vi "test_read-nmea-data2.vi"() -> ()   [LabVIEW 2019] (continued)
205,26,72,03,209,,1*76\n\t\n15:11:25.53\tF9P\t$GLGSV,2,2,08,77,01,326,,84,20,122,08,85,70,065,25,86,36,330,,1*74\n\t\n15:11:25.55\tF9P\t$GLGSV,2,1,08,69,12,031,,70,72,041,,71,51,205,24,72,03,209,,3*76\n\t\n15:11:25.57\tF9P\t$GLGSV,2,2,08,77,01,326,,84,20,122,18,85,70,065,21,86,36,330,,3*73\n\t\n15:11:25.59\tF9P\t$GAGSV,2,1,08,02,08,297,09,04,66,118,29,09,32,193,26,11,71,358,24,7*79\n\t\n15:11:25.61\tF9P\t$GAGSV,2,2,08,12,40,102,26,19,26,045,17,25,09,249,,36,26,308,35,7*7D\n\t\n15:11:25.63\tF9P\t$GAGSV,2,1,08,02,08,297,,04,66,118,27,09,32,193,,11,71,358,,2*79\n\t\n15:11:25.65\tF9P\t$GAGSV,2,2,08,12,40,102,,19,26,045,,25,09,249,,36,26,308,,2*7C\n\t\n15:11:25.67\tF9P\t$GBGSV,1,1,03,11,50,132,26,14,87,127,23,33,60,219,24,1*41\n\t\n15:11:25.69\tF9P\t$GBGSV,1,1,03,11,50,132,30,14,87,127,,33,60,219,,3*43\n\t\n15:11:25.71\tF9P\t$GNGLL,3723.53368,N,12656.90596,E,061127.00,A,A*7F\n\t\n15:11:25.73\tF9P\t\t\n15:11:25.75\tF9P\t\t\n15:11:25.77\tF9P\t\t\n15:11:25.79\tF9P\t\t\n15:11:25.81\tF9P\t\t\n15:11:25.83\tF9P\t\t\n15:11:25.85\tF9P\t\t\n15:11:25.87\tF9P\t\t\n15:11:25.89\tF9P\t\t\n15:11:25.91\tF9P\t\t\n15:11:25.93\tF9P\t\t\n15:11:25.95\tF9P\t\t\n15:11:25.97\tF9P\t\t\n15:11:25.99\tF9P\t\t\n15:11:26.01\tF9P\t\t\n15:11:26.03\tF9P\t\t\n15:11:26.05\tF9P\t\t\n15:11:26.07\tF9P\t\t\n15:11:26.09\tF9P\t\t\n15:11:26.11\tF9P\t\t\n15:11:26.13\tF9P\t\t\n15:11:26.15\tF9P\t\t\n15:11:26.17\tF9P\t\t\n15:11:26.19\tF9P\t\t\n15:11:26.21\tF9P\t\t\n15:11:26.23\tF9P\t\t\n15:11:26.25\tF9P\t$GNRMC,061128.00,A,3723.53331,N,12656.90644,E,1.898,132.24,250720,,,A,V*01\n\t\n15:11:26.27\tF9P\t$GNVTG,132.24,T,,M,1.898,N,3.516,K,A*2C\n\t\n15:11:26.29\tF9P\t$GNGGA,061128.00,3723.53331,N,12656.90644,E,1,12,0.72,35.9,M,18.5,M,,*70\n\t\n15:11:26.32\tF9P\t$GNGSA,A,3,12,06,19,05,17,09,04,02,,,,,1.36,0.72,1.15,1*04\n\t\n15:11:26.34\tF9P\t$GNGSA,A,3,85,71,84,,,,,,,,,,1.36,0.72,1.15,2*01\n\t\n15:11:26.36\tF9P\t$GNGSA,A,3,36,19,11,04,09,12,,,,,,,1.36,0.72,1.15,3*04\n\t\n15:11:26.38\tF9P\t$GNGSA,A,3,14,11,33,,,,,,,,,,1.36,0.72,1.15,4*05\n\t\n15:11:26.40\tF9P\t$GPGSV,3,1,09,02,54,318,30,04,18,044,18,05,37,247,19,06,64,047,30,1*6D\n\t\n15:11:26.42\tF9P\t$GPGSV,3,2,09,09,45,074,31,12,24,277,22,17,33,153,28,19,53,157,31,1*66\n\t\n15:11:26.44\tF9P\t$GPGSV,3,3,09,25,12,307,16,1*5A\n\t\n15:11:26.46\tF9P\t$GPGSV,3,1,09,02,54,318,,04,18,044,,05,37,247,19,06,64,047,29,6*68\n\t\n15:11:26.48\tF9P\t$GPGSV,3,2,09,09,45,074,31,12,24,277,,17,33,153,23,19,53,157,,6*68\n\t\n15:11:26.50\tF9P\t$GPGSV,3,3,09,25,12,307,,6*5A\n\t\n15:11:26.52\tF9P\t$GLGSV,2,1,08,69,12,031,,70,72,041,,71,51,205,26,72,03,209,,1*76\n\t\n15:11:26.54\tF9P\t$GLGSV,2,2,08,77,01,326,,84,20,122,10,85,70,065,37,86,36,330,,1*7E\n\t\n15:11:26.56\tF9P\t$GLGSV,2,1,08,69,12,031,,70,72,041,,71,51,205,24,72,03,209,,3*76\n\t\n15:11:26.58\tF9P\t$GLGSV,2,2,08,77,01,326,,84,20,122,20,85,70,065,22,86,36,330,,3*7B\n\t\n15:11:26.60\tF9P\t$GAGSV,2,1,08,02,08,297,09,04,66,118,28,09,32,193,26,11,71,358,24,7*78\n\t\n15:11:26.62\tF9P\t$GAGSV,2,2,08,12,40,102,24,19,26,045,14,25,09,249,,36,26,308,30,7*79\n\t\n15:11:26.64\tF9P\t$GAGSV,2,1,08,02,08,297,,04,66,118,27,09,32,193,,11,71,358,,2*79\n\t\n15:11:26.66\tF9P\t$GAGSV,2,2,08,12,40,102,,19,26,045,,25,09,249,,36,26,308,,2*7C\n\t\n15:11:26.68\tF9P\t$GBGSV,1,1,03,11,50,132,28,14,87,127,23,33,60,219,26,1*4D\n\t\n15:11:26.70\tF9P\t$GBGSV,1,1,03,11,50,132,,14,87,127,,33,60,219,,3*40\n\t\n15:11:26.72\tF9P\t$GNGLL,3723.53331,N,12656.90644,E,061128.00,A,A*70\n\t\n15:11:26.74\tF9P\t\t\n15:11:26.76\tF9P\t\t\n15:11:26.78\tF9P\t\t\n15:11:26.80\tF9P\t\t\n15:11:26.82\tF9P\t\t\n15:11:26.84\tF9P\t\t\n15:11:26.86\tF9P\t\t\n15:11:26.88\tF9P\t\t\n15:11:26.90\tF9P\t\t\n15:11:26.92\tF9P\t\t\n15:11:26.94\tF9P\t\t\n15:11:26.96\tF9P\t\t\n15:11:26.98\tF9P\t\t\n15:11:27.00\tF9P\t\t\n15:11:27.02\tF9P\t\t\n15:11:27.04\tF9P\t\t\n15:11:27.06\tF9P\t\t\n15:11:27.08\tF9P\t\t\n15:11:27.10\tF9P\t\t\n15:11:27.12\tF9P\t\t\n15:11:27.14\tF9P\t\t\n15:11:27.16\tF9P\t\t\n15:11:27.18\tF9P\t\t\n15:11:27.20\tF9P\t\t\n15:11:27.22\tF9P\t\t\n15:11:27.24\tF9P\t\t\n15:11:27.26\tF9P\t$GNRMC,061129.00,A,3723.53261,N,12656.90690,E,1.894,136.64,250720,,,A,V*01\n\t\n15:11:27.28\tF9P\t$GNVTG,136.64,T,,M,1.894,N,3.507,K,A*20\n\t\n15:11:27.30\tF9P\t$GNGGA,061129.00,3723.53261,N,12656.90690,E,1,12,0.72,36.2,M,18.5,M,,*74\n\t\n15:11:27.32\tF9P\t$GNGSA,A,3,12,06,19,05,17,09,02,,,,,,1.36,0.72,1.15,1*00\n\t\n15:11:27.34\tF9P\t$GNGSA,A,3,85,71,84,,,,,,,,,,1.36,0.72,1.15,2*01\n\t\n15:11:27.36\tF9P\t$GNGSA,A,3,36,19,11,04,09,12,,,,,,,1.36,0.72,1.15,3*04\n\t\n15:11:27.38\tF9P\t$GNGSA,A,3,14,11,33,,,,,,,,,,1.36,0.72,1.15,4*05\n\t\n15:11:27.40\tF9P\t$GPGSV,3,1,09,02,54,318,25,04,18,044,,05,37,247,22,06,64,047,29,1*60\n\t\n15:11:27.42\tF9P\t$GPGSV,3,2,09,09,45,074,32,12,24,277,22,17,33,153,32,19,53,157,39,1*66\n\t\n15:11:27.44\tF9P\t$GPGSV,3,3,09,25,12,307,17,1*5B\n\t\n15:11:27.46\tF9P\t$GPGSV,3,1,09,02,54,318,,04,18,044,,05,37,247,19,06,64,047,32,6*62\n\t\n15:11:27.48\tF9P\t$GPGSV,3,2,09,09,45,074,28,12,24,277,,17,33,153,24,19,53,157,,6*67\n\t\n15:11:27.50\tF9P\t$GPGSV,3,3,09,25,12,307,,6*5A\n\t\n15:11:27.52\tF9P\t$GLGSV,2,1,08,69,12,031,,70,72,041,,71,51,205,37,72,03,209,,1*76\n\t\n15:11:27.54\tF9P\t$GLGSV,2,2,08,77,01,326,,84,20,122,10,85,70,065,30,86,36,330,,1*79\n\t\n15:11:27.56\tF9P\t$GLGSV,2,1,08,69,12,031,,70,72,041,,71,51,205,31,72,03,209,,3*72\n\t\n15:11:27.58\tF9P\t$GLGSV,2,2,08,77,01,326,,84,20,122,19,85,70,065,30,86,36,330,,3*72\n\t\n15:11:27.60\tF9P\t$GAGSV,2,1,08,02,08,297,09,04,66,118,26,09,32,193,31,11,71,358,24,7*70\n\t\n15:11:27.62\tF9P\t$GAGSV,2,2,08,12,40,102,24,19,26,045,12,25,09,249,,36,26,308,28,7*76\n\t\n15:11:27.64\tF9P\t$GAGSV,2,1,08,02,08,297,,04,66,118,27,09,32,193,,11,71,358,,2*79\n\t\n15:11:27.66\tF9P\t$GAGSV,2,2,08,12,40,102,,19,26,045,,25,09,249,,36,26,308,,2*7C\n\t\n15:11:27.68\tF9P\t$GBGSV,1,1,03,11,50,132,27,14,87,127,31,33,60,219,31,1*47\n\t\n15:11:27.70\tF9P\t$GBGSV,1,1,03,11,50,132,27,14,87,127,,33,60,219,,3*45\n\t\n15:11:27.72\tF9P\t$GNGLL,3723.53261,N,12656.90690,E,061129.00,A,A*7C\n\t\n15:11:27.74\tF9P\t\t\n15:11:27.76\tF9P\t\t\n15:11:27.78\tF9P\t\t\n15:11:27.80\tF9P\t\t\n15:11:27.82\tF9P\t\t\n15:11:27.84\tF9P\t\t\n15:11:27.86\tF9P\t\t\n15:11:27.88\tF9P\t\t\n15:11:27.90\tF9P\t\t\n15:11:27.92\tF9P\t\t\n15:11:27.94\tF9P\t\t\n15:11:27.96\tF9P\t\t\n15:11:27.98\tF9P\t\t\n15:11:28.00\tF9P\t\t\n15:11:28.02\tF9P\t\t\n15:11:28.04\tF9P\t\t\n15:11:28.06\tF9P\t\t\n15:11:28.08\tF9P\t\t\n15:11:28.10\tF9P\t\t\n15:11:28.12\tF9P\t\t\n15:11:28.14\tF9P\t\t\n15:11:28.16\tF9P\t\t\n15:11:28.18\tF9P\t\t\n15:11:28.20\tF9P\t\t\n15:11:28.22\tF9P\t\t\n15:11:28.24\tF9P\t\t\n15:11:28.26\tF9P\t$GNRMC,061130.00,A,3723.53163,N,12656.90719,E,2.333,141.66,250720,,,A,V*0F\n\t\n15:11:28.28\tF9P\t$GNVTG,141.66,T,,M,2.333,N,4.322,K,A*21\n\t\n15:11:28.30\tF9P\t$GNGGA,061130.00,3723.53163,N,12656.90719,E,1,12,0.72,35.9,M,18.5,M,,*75\n\t\n15:11:28.32\tF9P\t$GNGSA,A,3,12,06,19,05,17,09,02,,,,,,1.36,0.72,1.15,1*00\n\t\n15:11:28.34\tF9P\t$GNGSA,A,3,85,71,84,,,,,,,,,,1.36,0.72,1.15,2*01\n\t\n15:11:28.36\tF9P\t$GNGSA,A,3,36,19,11,04,09,12,,,,,,,1.36,0.72,1.15,3*04\n\t\n15:11:28.38\tF9P\t$GNGSA,A,3,14,11,33,,,,,,,,,,1.36,0.72,1.15,4*05\n\t\n15:11:28.40\tF9P\t$GPGSV,3,1,09,02,54,318,32,04,18,044,,05,37,247,25,06,64,047,30,1*69\n\t\n15:11:28.42\tF9P\t$GPGSV,3,2,09,09,45,074,27,12,24,277,23,17,33,153,39,19,53,157,29,1*69\n\t\n15:11:28.44\tF9P\t$GPGSV,3,3,09,25,12,307,16,1*5A\n\t\n15:11:28.46\tF9P\t$GPGSV,3,1,09,02,54,318,,04,18,044,,05,37,247,17,06,64,047,27,6*68\n\t\n15:11:28.48\tF9P\t$GPGSV,3,2,09,09,45,074,26,12,24,277,,17,33,153,24,19,53,157,,6*69\n\t\n15:11:28.50\tF9P\t$GPGSV,3,3,09,25,12,307,,6*5A\n\t\n15:11:28.52\tF9P\t$GLGSV,2,1,08,69,12,031,,70,72,041,,71,51,205,32,72,03,209,,1*73\n\t\n15:11:28.54\tF9P\t$GLGSV,2,2,08,77,01,326,,84,20,122,16,85,70,065,24,86,36,330,,1*7A\n\t\n15:11:28.56\tF9P\t$GLGSV,2,1,08,69,12,031,,70,72,041,,71,51,205,24,72,03,209,,3*76\n\t\n15:11:28.58\tF9P\t$GLGSV,2,2,08,77,01,326,,84,20,122,17,85,70,065,23,86,36,330,,3*7E\n\t\n15:11:28.60\tF9P\t$GAGSV,2,1,08,02,08,297,11,04,66,118,30,09,32,193,26,11,71,358,23,7*7F\n\t\n15:11:28.62\tF9P\t$GAGSV,2,2,08,12,40,102,24,19,26,045,10,25,09,249,,36,26,308,29,7*75\n\t\n15:11:28.64\tF9P\t$GAGSV,2,1,08,02,08,297,,04,66,118,30,09,32,193,32,11,71,358,,2*7E\n\t\n15:11:28.66\tF9P\t$GAGSV,2,2,08,12,40,102,26,19,26,045,,25,09,249,,36,26,308,,2*78\n\t\n15:11:28.68\tF9P\t$GBGSV,1,1,03,11,50,132,27,14,87,127,26,33,60,219,36,1*46\n\t\n15:11:28.70\tF9P\t$GBGSV,1,1,03,11,50,132,27,14,87,127,,33,60,219,,3*45\n\t\n15:11:28.72\tF9P\t$GNGLL,3723.53163,N,12656.90719,E,061130.00,A,A*75\n\t\n15:11:28.74\tF9P\t\t\n15:11:28.76\tF9P\t\t\n15:11:28.78\tF9P\t\t\n15:11:28.80\tF9P\t\t\n15:11:28.82\tF9P\t\t\n15:11:28.84\tF9P\t\t\n15:11:28.86\tF9P\t\t\n15:11:28.88\tF9P\t\t\n15:11:28.90\tF9P\t\t\n15:11:28.92\tF9P\t\t\n15:11:28.94\tF9P\t\t\n15:11:28.96\tF9P\t\t\n15:11:28.98\tF9P\t\t\n15:11:29.00\tF9P\t\t\n15:11:29.02\tF9P\t\t\n15:11:29.04\tF9P\t\t\n15:11:29.06\tF9P\t\t\n15:11:29.08\tF9P\t\t\n15:11:29.10\tF9P\t\t\n15:11:29.12\tF9P\t\t\n15:11:29.14\tF9P\t\t\n15:11:29.16\tF9P\t\t\n15:11:29.18\tF9P\t\t\n15:11:29.20\tF9P\t\t\n15:11:29.22\tF9P\t\t\n15:11:29.24\tF9P\t$GNRMC,061131.00,A,3723.53091,N,12656.90746,E,2.306,147.77,250720,,,A,V*08\n\t\n15:11:29.26\tF9P\t$GNVTG,147.77,T,,M,2.306,N,4.271,K,A*26\n\t\n15:11:29.28\tF9P\t$GNGGA,061131.00,3723.53091,N,12656.90746,E,1,12,0.79,35.8,M,18.5,M,,*78\n\t\n15:11:29.30\tF9P\t$GNGSA,A,3,12,06,19,05,17,09,02,,,,,,1.50,0.79,1.27,1*0A\n\t\n15:11:29.32\tF9P\t$GNGSA,A,3,85,71,84,,,,,,,,,,1.50,0.79,1.27,2*0B\n\t\n15:11:29.34\tF9P\t$GNGSA,A,3,36,19,11,04,09,12,,,,,,,1.50,0.79,1.27,3*0E\n\t\n15:11:29.36\tF9P\t$GNGSA,A,3,14,11,33,,,,,,,,,,1.50,0.79,1.27,4*0F\n\t\n15:11:29.38\tF9P\t$GPGSV,3,1,09,02,54,318,31,04,18,044,18,05,37,247,31,06,64,047,34,1*62\n\t\n15:11:29.40\tF9P\t$GPGSV,3,2,09,09,45,074,31,12,24,277,23,17,33,153,34,19,53,157,32,1*69\n\t\n15:11:29.42\tF9P\t$GPGSV,3,3,09,25,12,307,15,1*59\n\t\n15:11:29.44\tF9P\t$GPGSV,3,1,09,02,54,318,,04,18,044,,05,37,247,15,06,64,047,25,6*68\n\t\n15:11:29.46\tF9P\t$GPGSV,3,2,09,09,45,074,27,12,24,277,,17,33,153,34,19,53,157,,6*69\n\t\n15:11:29.48\tF9P\t$GPGSV,3,3,09,25,12,307,,6*5A\n\t\n15:11:29.50\tF9P\t$GLGSV,2,1,08,69,12,031,,70,72,041,,71,51,205,32,72,03,209,,1*73\n\t\n15:11:29.52\tF9P\t$GLGSV,2,2,08,77,01,326,,84,20,122,10,85,70,065,30,86,36,330,,1*79\n\t\n15:11:29.54\tF9P\t$GLGSV,2,1,08,69,12,031,,70,72,041,,71,51,205,24,72,03,209,,3*76\n\t\n15:11:29.56\tF9P\t$GLGSV,2,2,08,77,01,326,,84,20,122,13,85,70,065,22,86,36,330,,3*7B\n\t\n15:11:29.58\tF9P\t$GAGSV,2,1,08,02,08,297,09,04,66,118,30,09,32,193,35,11,71,358,25,7*72\n\t\n15:11:29.60\tF9P\t$GAGSV,2,2,08,12,40,102,24,19,26,045,15,25,09,249,,36,26,308,31,7*79\n\t\n15:11:29.62\tF9P\t$GAGSV,2,1,08,02,08,297,,04,66,118,30,09,32,193,26,11,71,358,,2*7B\n\t\n15:11:29.64\tF9P\t$GAGSV,2,2,08,12,40,102,25,19,26,045,,25,09,249,,36,26,308,,2*7B\n\t\n15:11:29.66\tF9P\t$GBGSV,1,1,03,11,50,132,26,14,87,127,26,33,60,219,33,1*42\n\t\n15:11:29.68\tF9P\t$GBGSV,1,1,03,11,50,132,,14,87,127,,33,60,219,,3*40\n\t\n15:11:29.70\tF9P\t$GNGLL,3723.53091,N,12656.90746,E,061131.00,A,A*72\n\t\n15:11:29.72\tF9P\t\t\n15:11:29.74\tF9P\t\t\n15:11:29.76\tF9P\t\t\n15:11:29.78\tF9P\t\t\n15:11:29.80\tF9P\t\t\n15:11:29.82\tF9P\t\t\n15:11:29.84\tF9P\t\t\n15:11:29.86\tF9P\t\t\n15:11:29.88\tF9P\t\t\n15:11:29.90\tF9P\t\t\n15:11:29.92\tF9P\t\t\n15:11:29.94\tF9P\t\t\n15:11:29.96\tF9P\t\t\n15:11:29.98\tF9P\t\t\n15:11:30.00\tF9P\t\t\n15:11:30.02\tF9P\t\t\n15:11:30.04\tF9P\t\t\n15:11:30.06\tF9P\t\t\n15:11:30.08\tF9P\t\t\n15:11:30.10\tF9P\t\t\n15:11:30.12\tF9P\t\t\n15:11:30.14\tF9P\t\t\n15:11:30.16\tF9P\t\t\n15:11:30.18\tF9P\t\t\n15:11:30.20\tF9P\t\t\n15:11:30.22\tF9P\t\t\n15:11:30.24\tF9P\t\t\n15:11:30.26\tF9P\t$GNRMC,061132.00,A,3723.53020,N,12656.90826,E,2.392,137.11,250720,,,A,V*02\n\t\n15:11:30.28\tF9P\t$GNVTG,137.11,T,,M,2.392,N,4.430,K,A*2F\n\t\n15:11:30.30\tF9P\t$GNGGA,061132.00,3723.53020,N,12656.90826,E,1,12,0.68,35.3,M,18.5,M,,*73\n\t\n15:11:30.32\tF9P\t$GNGSA,A,3,12,06,19,05,17,09,02,,,,,,1.27,0.68,1.08,1*07\n\t\n15:11:30.34\tF9P\t$GNGSA,A,3,85,71,84,,,,,,,,,,1.27,0.68,1.08,2*06\n\t\n15:11:30.36\tF9P\t$GNGSA,A,3,36,19,11,04,09,12,,,,,,,1.27,0.68,1.08,3*03\n\t\n15:11:30.38\tF9P\t$GNGSA,A,3,14,11,33,,,,,,,,,,1.27,0.68,1.08,4*02\n\t\n15:11:30.40\tF9P\t$GPGSV,3,1,09,02,54,318,35,04,18,044,19,05,37,247,24,06,64,047,39,1*6E\n\t\n15:11:30.42\tF9P\t$GPGSV,3,2,09,09,45,074,33,12,24,277,29,17,33,153,38,19,53,157,36,1*69\n\t\n15:11:30.44\tF9P\t$GPGSV,3,3,09,25,12,307,16,1*5A\n\t\n15:11:30.46\tF9P\t$GPGSV,3,1,09,02,54,318,,04,18,044,,05,37,247,,06,64,047,23,6*6A\n\t\n15:11:30.48\tF9P\t$GPGSV,3,2,09,09,45,074,27,12,24,277,,17,33,153,22,19,53,157,,6*6E\n\t\n15:11:30.50\tF9P\t$GPGSV,3,3,09,25,12,307,,6*5A\n\t\n15:11:30.52\tF9P\t$GLGSV,2,1,08,69,12,031,,70,72,041,,71,51,205,39,72,03,209,,1*78\n\t\n15:11:30.54\tF9P\t$GLGSV,2,2,08,77,01,326,,84,20,122,11,85,70,065,30,86,36,330,,1*78\n\t\n15:11:30.56\tF9P\t$GLGSV,2,1,08,69,12,031,,70,72,041,,71,51,205,31,72,03,209,,3*72\n\t\n15:11:30.58\tF9P\t$GLGSV,2,2,08,77,01,326,,84,20,122,16,85,70,065,21,86,36,330,,3*7D\n\t\n15:11:30.60\tF9P\t$GAGSV,2,1,08,02,08,297,11,04,66,118,30,09,32,193,28,11,71,358,21,7*73\n\t\n15:11:30.62\tF9P\t$GAGSV,2,2,08,12,40,102,23,19,26,045,10,25,09,249,,36,26,308,32,7*78\n\t\n15:11:30.64\tF9P\t$GAGSV,2,1,08,02,08,297,,04,66,118,25,09,32,193,25,11,71,358,,2*7C\n\t\n15:11:30.66\tF9P\t$GAGSV,2,2,08,12,40,102,25,19,26,045,,25,09,249,,36,26,308,,2*7B\n\t\n15:11:30.68\tF9P\t$GBGSV,1,1,03,11,50,132,26,14,87,127,30,33,60,219,35,1*43\n\t\n15:11:30.70\tF9P\t$GBGSV,1,1,03,11,50,132,27,14,87,127,,33,60,219,,3*45\n\t\n15:11:30.72\tF9P\t$GNGLL,3723.53020,N,12656.90826,E,061132.00,A,A*72\n\t\n15:11:30.74\tF9P\t\t\n15:11:30.76\tF9P\t\t\n15:11:30.78\tF9P\t\t\n15:11:30.80\tF9P\t\t\n15:11:30.82\tF9P\t\t\n15:11:30.84\tF9P\t\t\n15:11:30.86\tF9P\t\t\n15:11:30.88\tF9P\t\t\n15:11:30.90\tF9P\t\t\n15:11:30.92\tF9P\t\t\n15:11:30.94\tF9P\t\t\n15:11:30.96\tF9P\t\t\n15:11:30.98\tF9P\t\t\n15:11:31.00\tF9P\t\t\n15:11:31.02\tF9P\t\t\n15:11:31.04\tF9P\t\t\n15:11:31.06\tF9P\t\t\n15:11:31.08\tF9P\t\t\n15:11:31.10\tF9P\t\t\n15:11:31.12\tF9P\t\t\n15:11:31.14\tF9P\t\t\n15:11:31.16\tF9P\t\t\n15:11:31.18\tF9P\t\t\n15:11:31.20\tF9P\t\t\n15:11:31.22\tF9P\t\t\n15:11:31.24\tF9P\t$GNRMC,061133.00,A,3723.52963,N,12656.90859,E,2.005,138.73,250720,,,A,V*02\n\t\n15:11:31.26\tF9P\t$GNVTG,138.73,T,,M,2.005,N,3.714,K,A*2B\n\t\n15:11:31.28\tF9P\t$GNGGA,061133.00,3723.52963,N,12656.90859,E,1,12,0.72,35.3,M,18.5,M,,*7E\n\t\n15:11:31.30\tF9P\t$GNGSA,A,3,12,06,19,05,17,09,02,,,,,,1.36,0.72,1.15,1*00\n\t\n15:11:31.32\tF9P\t$GNGSA,A,3,85,71,84,,,,,,,,,,1.36,0.72,1.15,2*01\n\t\n15:11:31.34\tF9P\t$GNGSA,A,3,36,19,11,04,09,12,,,,,,,1.36,0.72,1.15,3*04\n\t\n15:11:31.36\tF9P\t$GNGSA,A,3,14,11,33,,,,,,,,,,1.36,0.72,1.15,4*05\n\t\n15:11:31.38\tF9P\t$GPGSV,3,1,09,02,54,318,35,04,18,044,18,05,37,247,24,06,64,047,38,1*6E\n\t\n15:11:31.40\tF9P\t$GPGSV,3,2,09,09,45,074,32,12,24,277,27,17,33,153,35,19,53,157,33,1*6E\n\t\n15:11:31.42\tF9P\t$GPGSV,3,3,09,25,12,307,17,1*5B\n\t\n15:11:31.44\tF9P\t$GPGSV,3,1,09,02,54,318,,04,18,044,,05,37,247,,06,64,047,21,6*68\n\t\n15:11:31.46\tF9P\t$GPGSV,3,2,09,09,45,074,27,12,24,277,,17,33,153,22,19,53,157,,6*6E\n\t\n15:11:31.48\tF9P\t$GPGSV,3,3,09,25,12,307,,6*5A\n\t\n15:11:31.50\tF9P\t$GLGSV,2,1,08,69,12,031,,70,71,039,,71,51,205,32,72,03,209,,1*7F\n\t\n15:11:31.52\tF9P\t$GLGSV,2,2,08,77,01,326,,84,20,122,17,85,70,065,30,86,36,330,,1*7E\n\t\n15:11:31.54\tF9P\t$GLGSV,2,1,08,69,12,031,,70,71,039,,71,51,205,27,72,03,209,,3*79\n\t\n15:11:31.56\tF9P\t$GLGSV,2,2,08,77,01,326,,84,20,122,15,85,70,065,22,86,36,330,,3*7D\n\t\n15:11:31.58\tF9P\t$GAGSV,2,1,08,02,08,297,10,04,66,118,29,09,32,193,31,11,71,358,29,7*7A\n\t\n15:11:31.60\tF9P\t$GAGSV,2,2,08,12,40,102,23,19,26,045,10,25,09,249,,36,26,308,37,7*7D\n\t\n15:11:31.62\tF9P\t$GAGSV,2,1,08,02,08,297,,04,66,118,24,09,32,193,25,11,71,358,,2*7D\n\t\n15:11:31.64\tF9P\t$GAGSV,2,2,08,12,40,102,26,19,26,045,,25,09,249,,36,26,308,,2*78\n\t\n15:11:31.66\tF9P\t$GBGSV,1,1,03,11,50,132,31,14,87,127,25,33,60,219,31,1*45\n\t\n15:11:31.68\tF9P\t$GBGSV,1,1,03,11,50,132,26,14,87,127,,33,60,219,,3*44\n\t\n15:11:31.70\tF9P\t$GNGLL,3723.52963,N,12656.90859,E,061133.00,A,A*74\n\t\n15:11:31.72\tF9P\t\t\n15:11:31.74\tF9P\t\t\n15:11:31.76\tF9P\t\t\n15:11:31.78\tF9P\t\t\n15:11:31.80\tF9P\t\t\n15:11:31.82\tF9P\t\t\n15:11:31.84\tF9P\t\t\n15:11:31.86\tF9P\t\t\n15:11:31.88\tF9P\t\t\n15:11:31.90\tF9P\t\t\n15:11:31.92\tF9P\t\t\n15:11:31.94\tF9P\t\t\n15:11:31.96\tF9P\t\t\n15:11:31.98\tF9P\t\t\n15:11:32.00\tF9P\t\t\n15:11:32.02\tF9P\t\t\n15:11:32.04\tF9P\t\t\n15:11:32.06\tF9P\t\t\n15:11:32.08\tF9P\t\t\n15:11:32.10\tF9P\t\t\n15:11:32.12\tF9P\t\t\n15:11:32.14\tF9P\t\t\n15:11:32.16\tF9P\t\t\n15:11:32.18\tF9P\t\t\n15:11:32.20\tF9P\t\t\n15:11:32.22\tF9P\t\t\n15:11:32.24\tF9P\t\t\n15:11:32.26\tF9P\t$GNRMC,061134.00,A,3723.52948,N,12656.90973,E,2.314,119.55,250720,,,A,V*01\n\t\n15:11:32.28\tF9P\t$GNVTG,119.55,T,,M,2.314,N,4.285,K,A*25\n\t\n15:11:32.30\tF9P\t$GNGGA,061134.00,3723.52948,N,12656.90973,E,1,12,0.72,34.5,M,18.5,M,,*7E\n\t\n15:11:32.32\tF9P\t$GNGSA,A,3,12,06,19,05,17,09,02,,,,,,1.36,0.72,1.15,1*00\n\t\n15:11:32.34\tF9P\t$GNGSA,A,3,85,71,84,,,,,,,,,,1.36,0.72,1.15,2*01\n\t\n15:11:32.36\tF9P\t$GNGSA,A,3,36,19,11,04,09,12,,,,,,,1.36,0.72,1.15,3*04\n\t\n15:11:32.38\tF9P\t$GNGSA,A,3,14,11,33,,,,,,,,,,1.36,0.72,1.15,4*05\n\t\n15:11:32.40\tF9P\t$GPGSV,3,1,09,02,54,318,39,04,18,044,27,05,37,247,25,06,64,047,47,1*67\n\t\n15:11:32.42\tF9P\t$GPGSV,3,2,09,09,45,074,43,12,24,277,28,17,33,153,36,19,53,157,35,1*62\n\t\n15:11:32.44\tF9P\t$GPGSV,3,3,09,25,12,307,18,1*54\n\t\n15:11:32.46\tF9P\t$GPGSV,3,1,09,02,54,318,,04,18,044,,05,37,247,,06,64,047,20,6*69\n\t\n15:11:32.48\tF9P\t$GPGSV,3,2,09,09,45,074,25,12,24,277,,17,33,153,23,19,53,157,,6*6D\n\t\n15:11:32.50\tF9P\t$GPGSV,3,3,09,25,12,307,,6*5A\n\t\n15:11:32.52\tF9P\t$GLGSV,2,1,08,69,12,031,,70,71,039,,71,52,205,34,72,03,209,,1*7A\n\t\n15:11:32.54\tF9P\t$GLGSV,2,2,08,77,01,326,,84,20,122,15,85,70,065,37,86,36,330,,1*7B\n\t\n15:11:32.56\tF9P\t$GLGSV,2,1,08,69,12,031,,70,71,039,,71,52,205,25,72,03,209,,3*78\n\t\n15:11:32.58\tF9P\t$GLGSV,2,2,08,77,01,326,,84,20,122,15,85,70,065,23,86,36,330,,3*7C\n\t\n15:11:32.60\tF9P\t$GAGSV,2,1,08,02,08,297,07,04,66,118,32,09,32,193,27,11,71,358,34,7*7D\n\t\n15:11:32.62\tF9P\t$GAGSV,2,2,08,12,40,102,30,19,26,045,12,25,09,249,,36,26,308,30,7*7A\n\t\n15:11:32.64\tF9P\t$GAGSV,2,1,08,02,08,297,,04,66,118,,09,32,193,23,11,71,358,,2*7D\n\t\n15:11:32.66\tF9P\t$GAGSV,2,2,08,12,40,102,,19,26,045,,25,09,249,,36,26,308,,2*7C\n\t\n15:11:32.68\tF9P\t$GBGSV,1,1,03,11,50,132,30,14,87,127,26,33,60,219,31,1*47\n\t\n15:11:32.70\tF9P\t$GBGSV,1,1,03,11,50,132,27,14,87,127,32,33,60,219,,3*44\n\t\n15:11:32.72\tF9P\t$GNGLL,3723.52948,N,12656.90973,E,061134.00,A,A*73\n\t\n15:11:32.74\tF9P\t\t\n15:11:32.76\tF9P\t\t\n15:11:32.78\tF9P\t\t\n15:11:32.80\tF9P\t\t\n15:11:32.82\tF9P\t\t\n15:11:32.84\tF9P\t\t\n15:11:32.86\tF9P\t\t\n15:11:32.88\tF9P\t\t\n15:11:32.90\tF9P\t\t\n15:11:32.92\tF9P\t\t\n15:11:32.94\tF9P\t\t\n15:11:32.96\tF9P\t\t\n15:11:32.98\tF9P\t\t\n15:11:33.00\tF9P\t\t\n15:11:33.02\tF9P\t\t\n15:11:33.04\tF9P\t\t\n15:11:33.06\tF9P\t\t\n15:11:33.08\tF9P\t\t\n15:11:33.10\tF9P\t\t\n15:11:33.12\tF9P\t\t\n15:11:33.14\tF9P\t\t\n15:11:33.16\tF9P\t\t\n15:11:33.18\tF9P\t\t\n15:11:33.20\tF9P\t\t\n15:11:33.22\tF9P\t\t\n15:11:33.24\tF9P\t$GNRMC,061135.00,A,3723.52856,N,12656.91091,E,4.233,127.22,250720,,,A,V*05\n\t\n15:11:33.26\tF9P\t$GNVTG,127.22,T,,M,4.233,N,7.840,K,A*2A\n\t\n15:11:33.28\tF9P\t$GNGGA,061135.00,3723.52856,N,12656.91091,E,1,12,0.72,33.5,M,18.5,M,,*72\n\t\n15:11:33.30\tF9P\t$GNGSA,A,3,12,06,19,05,17,09,04,02,,,,,1.36,0.72,1.15,1*04\n\t\n15:11:33.32\tF9P\t$GNGSA,A,3,85,71,84,,,,,,,,,,1.36,0.72,1.15,2*01\n\t\n15:11:33.34\tF9P\t$GNGSA,A,3,36,19,11,04,09,12,,,,,,,1.36,0.72,1.15,3*04\n\t\n15:11:33.36\tF9P\t$GNGSA,A,3,14,11,33,,,,,,,,,,1.36,0.72,1.15,4*05\n\t\n15:11:33.38\tF9P\t$GPGSV,3,1,09,02,54,318,27,04,18,044,26,05,37,247,24,06,64,047,30,1*68\n\t\n15:11:33.40\tF9P
